vi "Test B.vi"(1 "board image":T1) -> (0 "pass?":T2)   [LabVIEW 2023]
doc: "Test an elite DAQ board image."
uses:
  Common/Pass Fail Boolean.ctl
  Common/Board Image.ctl
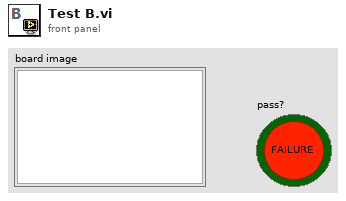
[diagram p1: front panel]
types:
  T1 = typedef "Board Image.ctl" = picture
  T2 = typedef "Pass Fail Boolean.ctl" = bool
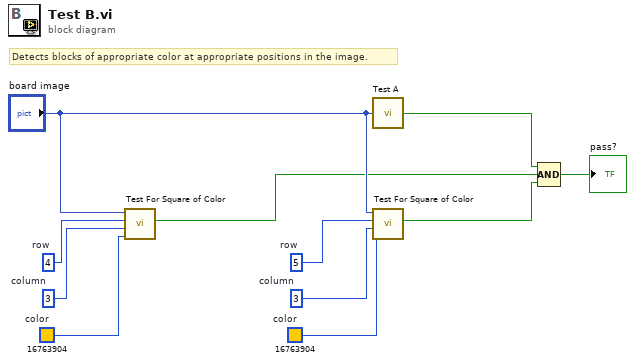
[diagram p0: block diagram]
diagram:
  w7 = i16 3  # column
  w6 = i16 5  # row
  w8 = u32 16763904  # color
  w10 = i16 3  # column
  w11 = i16 4  # row
  w9 = u32 16763904  # color
  # "Detects blocks of appropriate color at appropriate positions in the image."
  n1 = call "Test For Square of Color.vi"("color"=w9, "column"=w10, "row"=w11, "board image"="board image") -> ("pass?"=w3:T2)  [unwired: 7 in]
  n2 = call "Test A.vi"("board image"="board image") -> ("Pass?"=w4:T2)
  n3 = call "Test For Square of Color.vi"("color"=w8, "column"=w7, "row"=w6, "board image"="board image") -> ("pass?"=w2:T2)  [unwired: 7 in]
  n4 = Compound Arithmetic op=AND(w4, w3, w2) -> (→"pass?":T2)
